vi "pl1000SetDo.vi"(8 "error in (no error)":errorcluster, 9 "DO Channel":i32, 10 "DO State":bool, 11 "pl1000 handle":i16) -> (0 "error out":errorcluster, 3 "pl1000 handle out":i16)   [LabVIEW 2016, in "pl1000.lvlib"]
uses:
  pl1000.lvlib
  pl1000.dll
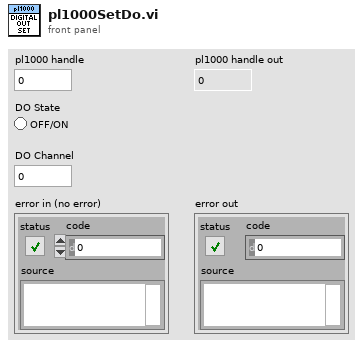
[diagram p1: front panel]
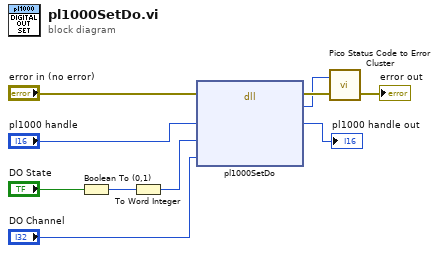
[diagram p0: block diagram]
diagram:
  n1 = Boolean To (0,1)(Boolean="DO State") -> (0, 1=w3:i16)
  n2 = To Word Integer(number=w3) -> (16bit integer=w2:i16)
  n3 = dll-call lib="pl1000.dll" fn="pl1000SetDo"(error in="error in (no error)", "handle"="pl1000 handle", "doValue"=w2, "doNo"="DO Channel") -> (error out=w8:errorcluster, "status"=w7:u32, "handle"=→"pl1000 handle out":i16)  [unwired: 4 in, 1 out]
  n4 = call "Pico Status Code to Error Cluster.vi"("error in"=w8, "PICO_STATUS"=w7) -> ("error out"=→"error out":errorcluster)  [unwired: 1 in]
